vi "initalize 4200(SubVI).vi"(0 "簇":T4={"initialize"=enum."SR830", "6221"={"6221 Resource"="GPIB0::24::INSTR", "Delta status"=FALSE, "电流|RMS(A)"=0.0}, "SR830+6221"={"source"=0, "Current(A)"=0.0, "阻抗(Ohm)"=0.0, "SR830 1"=FALSE, "SR830 2"=FALSE, "SR830 3"=FALSE, "SR830 4"=FALSE, "VISA 1"="", "VISA 2"="", "VISA 3"="", "VISA 4"="", "Reserve 1"=0, "Reserve 2"=-1, "Reserve 3"=-1, "Reserve 4"=-1, "Sensitivity 1"=-1, "Sensitivity 2"=-1, "Sensitivity 3"=-1, "Sensitivity 4"=-1, "量程入 1"=0, "量程入 2"=0, "量程入 3"=0, "量程入 4"=0}, "2400"={"2400"=FALSE, "VISA"="", "Output Level (0)"=1e-05, "Compliance  Level (0.1)"=10.0, "ch"=[]}, "ch"={"ch"=[], "current"=[], "change?"=[], "holding current\nwhen change ch?"=FALSE, "current offset"=[]}, "Instrument"={"limit"={"Field limit"=0.0, "Field rate limit"=0.0, "Temp limit"=0.0, "Temp low limit"=0.0, "Temp rate limit "=0.0}, "genarl"={"行数"=refnum, "编辑列表框？"=refnum, "列表框"=refnum, "camg 振荡状态"=refnum, "Aborting"=refnum, "数据文件"=refnum, "warning"=refnum, "vi路径"="", "Instrument Type"=enum."PPMS-Rotate"}, "cmag"={"TM620"="TCPIP0::192.168.1.5::4266::SOCKET", "M24C Resource"="GPIB0::24::INSTR", "4G supply"="", "Temp Status 24C"=refnum, "Temp"=refnum, "9T信号"=refnum, "4g supply status"=refnum, "in-plane"="", "out-plane"="", "in-plane signal"=FALSE, "out-plane signal"=FALSE, "in plane 信号"=refnum, "pzt volt"=refnum, "camg Rate"=refnum}, "lengtou2"={"750 visa"="", "750 rotate"="", "semaphore 340"=refnum, "semaphore 750"=refnum, "750 field status"=refnum, "Input (0:A) 340"=0, "340 Resource"="GPIB0::14::INSTR", "340 Status"=refnum, "Input (0:B) 340"=1, "Loop (0: 1)"=0, "Loop (1: 1)"=0, "TCP master instance"=refnum}, "lengtou"={"TCP master instance"=refnum, "335 Status"=refnum, "335 Resource "="GPIB0::24::INSTR", "Input (0:A) 335"=0, "Input (0:B) 335"=1, "Heater Output (1:1) 335"=1, "semaphore 335"=refnum}, "325 for test"={"quantum design"=refnum, "semaphore 325"=refnum, "325 Resource "="GPIB0::13::INSTR", "Input (0:A) 325"=0, "Heater Output (1:1) 325"=1, "325 Status"=refnum}}, "2614B"={"2614B chA"=FALSE, "2614B chB"=FALSE, "VISA"=""}, "33522b"={"33522b resource name"="GPIB0::16::INSTR", "零电压"=0.0, "最大电压"=148.0, "间隔"=4.0, "最小电压"=-48.0, "loop"=0.0, "压电陶瓷电压(Vpp)"=0.0}, "gating type"=enum."2614(daul)", "层数"=0, "行数"=0, "是否处理"=[], "current 2"=[], "StrainCell"={"RP100 resource name"="GPIB0::16::INSTR", "E4980 resource name"="GPIB0::16::INSTR", "RP100 Reset ?(True)"=TRUE, "Voltage1(V)"=0.0, "Voltage2(V)"=148.0, "interval"=4.0, "slew(V/s)"=-48.0}} {"Instrument"."325 for test"."Heater Output (1:1) 325" items=["1"=1, "2"=2]; "Instrument"."325 for test"."Input (0:A) 325" items=["A", "B"]; "Instrument"."lengtou"."Heater Output (1:1) 335" items=["1"=1, "2"=2]; "Instrument"."lengtou"."Input (0:B) 335" items=["A", "B"]; "Instrument"."lengtou"."Input (0:A) 335" items=["A", "B"]; "Instrument"."lengtou2"."Loop (1: 1)" items=["1", "2"]; "Instrument"."lengtou2"."Loop (0: 1)" items=["1", "2"]; "Instrument"."lengtou2"."Input (0:B) 340" items=["A", "B", "C", "D"]; "Instrument"."lengtou2"."Input (0:A) 340" items=["A", "B", "C", "D"]; "SR830+6221"."Sensitivity 4" items=["量程每次测量会判定", "量程不变为设定值"]; "SR830+6221"."Sensitivity 3" items=["Auto Reserve"=-1, "High Reserve"=0, "Normal"=1, "Low Noise"=2]; "SR830+6221"."Sensitivity 1" items=["Auto Reserve"=-1, "High Reserve"=0, "Normal"=1, "Low Noise"=2]; "SR830+6221"."Sensitivity 2" items=["Auto Reserve"=-1, "High Reserve"=0, "Normal"=1, "Low Noise"=2]; "SR830+6221"."Reserve 4" items=["量程每次测量会判定", "量程不变为设定值"]; "SR830+6221"."Reserve 3" items=["Auto Reserve"=-1, "High Reserve"=0, "Normal"=1, "Low Noise"=2]; "SR830+6221"."Reserve 2" items=["Auto Reserve"=-1, "High Reserve"=0, "Normal"=1, "Low Noise"=2]; "SR830+6221"."Reserve 1" items=["Auto Reserve"=-1, "High Reserve"=0, "Normal"=1, "Low Noise"=2]; "SR830+6221"."source" items=["SR830 1", "SR830 2", "SR830 3", "SR830 4"]}, 2 "字符串":string) -> (7 "输出簇":T4={"initialize"=enum."SR830", "6221"={"6221 Resource"="GPIB0::24::INSTR", "Delta status"=FALSE, "电流|RMS(A)"=0.0}, "SR830+6221"={"source"=0, "Current(A)"=0.0, "阻抗(Ohm)"=0.0, "SR830 1"=FALSE, "SR830 2"=FALSE, "SR830 3"=FALSE, "SR830 4"=FALSE, "VISA 1"="", "VISA 2"="", "VISA 3"="", "VISA 4"="", "Reserve 1"=0, "Reserve 2"=-1, "Reserve 3"=-1, "Reserve 4"=-1, "Sensitivity 1"=-1, "Sensitivity 2"=-1, "Sensitivity 3"=-1, "Sensitivity 4"=-1, "量程入 1"=0, "量程入 2"=0, "量程入 3"=0, "量程入 4"=0}, "2400"={"2400"=FALSE, "VISA"="", "Output Level (0)"=1e-05, "Compliance  Level (0.1)"=10.0, "ch"=[]}, "ch"={"ch"=[], "current"=[], "change?"=[], "holding current\nwhen change ch?"=FALSE, "current offset"=[]}, "Instrument"={"limit"={"Field limit"=0.0, "Field rate limit"=0.0, "Temp limit"=0.0, "Temp low limit"=0.0, "Temp rate limit "=0.0}, "genarl"={"行数"=refnum, "编辑列表框？"=refnum, "列表框"=refnum, "camg 振荡状态"=refnum, "Aborting"=refnum, "数据文件"=refnum, "warning"=refnum, "vi路径"="", "Instrument Type"=enum."PPMS-Rotate"}, "cmag"={"TM620"="TCPIP0::192.168.1.5::4266::SOCKET", "M24C Resource"="GPIB0::24::INSTR", "4G supply"="", "Temp Status 24C"=refnum, "Temp"=refnum, "9T信号"=refnum, "4g supply status"=refnum, "in-plane"="", "out-plane"="", "in-plane signal"=FALSE, "out-plane signal"=FALSE, "in plane 信号"=refnum, "pzt volt"=refnum, "camg Rate"=refnum}, "lengtou2"={"750 visa"="", "750 rotate"="", "semaphore 340"=refnum, "semaphore 750"=refnum, "750 field status"=refnum, "Input (0:A) 340"=0, "340 Resource"="GPIB0::14::INSTR", "340 Status"=refnum, "Input (0:B) 340"=1, "Loop (0: 1)"=0, "Loop (1: 1)"=0, "TCP master instance"=refnum}, "lengtou"={"TCP master instance"=refnum, "335 Status"=refnum, "335 Resource "="GPIB0::24::INSTR", "Input (0:A) 335"=0, "Input (0:B) 335"=1, "Heater Output (1:1) 335"=1, "semaphore 335"=refnum}, "325 for test"={"quantum design"=refnum, "semaphore 325"=refnum, "325 Resource "="GPIB0::13::INSTR", "Input (0:A) 325"=0, "Heater Output (1:1) 325"=1, "325 Status"=refnum}}, "2614B"={"2614B chA"=FALSE, "2614B chB"=FALSE, "VISA"=""}, "33522b"={"33522b resource name"="GPIB0::16::INSTR", "零电压"=0.0, "最大电压"=148.0, "间隔"=4.0, "最小电压"=-48.0, "loop"=0.0, "压电陶瓷电压(Vpp)"=0.0}, "gating type"=enum."2614(daul)", "层数"=0, "行数"=0, "是否处理"=[], "current 2"=[], "StrainCell"={"RP100 resource name"="GPIB0::16::INSTR", "E4980 resource name"="GPIB0::16::INSTR", "RP100 Reset ?(True)"=TRUE, "Voltage1(V)"=0.0, "Voltage2(V)"=148.0, "interval"=4.0, "slew(V/s)"=-48.0}} {"Instrument"."325 for test"."Heater Output (1:1) 325" items=["1"=1, "2"=2]; "Instrument"."325 for test"."Input (0:A) 325" items=["A", "B"]; "Instrument"."lengtou"."Heater Output (1:1) 335" items=["1"=1, "2"=2]; "Instrument"."lengtou"."Input (0:B) 335" items=["A", "B"]; "Instrument"."lengtou"."Input (0:A) 335" items=["A", "B"]; "Instrument"."lengtou2"."Loop (1: 1)" items=["1", "2"]; "Instrument"."lengtou2"."Loop (0: 1)" items=["1", "2"]; "Instrument"."lengtou2"."Input (0:B) 340" items=["A", "B", "C", "D"]; "Instrument"."lengtou2"."Input (0:A) 340" items=["A", "B", "C", "D"]; "SR830+6221"."Sensitivity 4" items=["量程每次测量会判定", "量程不变为设定值"]; "SR830+6221"."Sensitivity 3" items=["Auto Reserve"=-1, "High Reserve"=0, "Normal"=1, "Low Noise"=2]; "SR830+6221"."Sensitivity 1" items=["Auto Reserve"=-1, "High Reserve"=0, "Normal"=1, "Low Noise"=2]; "SR830+6221"."Sensitivity 2" items=["Auto Reserve"=-1, "High Reserve"=0, "Normal"=1, "Low Noise"=2]; "SR830+6221"."Reserve 4" items=["量程每次测量会判定", "量程不变为设定值"]; "SR830+6221"."Reserve 3" items=["Auto Reserve"=-1, "High Reserve"=0, "Normal"=1, "Low Noise"=2]; "SR830+6221"."Reserve 2" items=["Auto Reserve"=-1, "High Reserve"=0, "Normal"=1, "Low Noise"=2]; "SR830+6221"."Reserve 1" items=["Auto Reserve"=-1, "High Reserve"=0, "Normal"=1, "Low Noise"=2]; "SR830+6221"."source" items=["SR830 1", "SR830 2", "SR830 3", "SR830 4"]})   [LabVIEW 2019, in "initialize.lvlib"]
uses:
  initialize.lvlib
  ctl/config.ctl
  <vilib>/NI/Modbus Library/API/Master/Modbus Master.lvclass
  ctl/initialize.ctl
  ctl/Instrument.ctl
  ctl/limit.ctl
  ctl/warning.ctl
  ctl/Instrument Type.ctl
  ctl/335 state.ctl
  ctl/9T mag field stauts.ctl
  C:/Users/fuyang/Desktop/postdoctor/labview/labview-measure/lib/QDInstrument.dll
  lib/QDInstrument.dll
  ctl/Gating type.ctl
panel:
  out "Name array 2":string[](array[string])
  in  "SMU2(Ryx) Setup":T1={"Enable"=TRUE, "Source Mode"=enum."Voltage Source", "Compliance (V/A)"=0.1, "Source V/I (V/A)"=0.0, "Current Measurement Range\n(Limited Auto)"=9} {"Current Measurement Range\n(Limited Auto)" items=["1 pA (pre-Amp only)", "10 pA (pre-Amp only)", "100 pA (pre-Amp only)", "1 nA", "10 nA", "100 nA", "1 uA", "10 uA", "100 uA", "1 mA", "10 mA", "100 mA", "1 A (4210-SMU only)"]; "Source V/I (V/A)" min=-100.0 max=100.0 step=0.0001 format="%^.2e"; "Compliance (V/A)" min=-210.0 max=210.0 format="%_3e"}
  in  "SMU1(Rxx) Setup":T1={"Enable"=TRUE, "Source Mode"=enum."Voltage Source", "Compliance (V/A)"=0.1, "Source V/I (V/A)"=0.0, "Current Measurement Range\n(Limited Auto)"=9} {"Current Measurement Range\n(Limited Auto)" items=["1 pA (pre-Amp only)", "10 pA (pre-Amp only)", "100 pA (pre-Amp only)", "1 nA", "10 nA", "100 nA", "1 uA", "10 uA", "100 uA", "1 mA", "10 mA", "100 mA", "1 A (4210-SMU only)"]; "Source V/I (V/A)" min=-100.0 max=100.0 step=0.0001 format="%^.2e"; "Compliance (V/A)" min=-210.0 max=210.0 format="%_3e"}
  in  "Integration Time":i16(slide)=2 min=1 max=3 step=1 scale=1.0..3.0
  out "Name array":string[](array[string])
  out "SMU1 status":T2
  out "4200 GPIB address out":string="1::17"
  out "error out":errorcluster
  in  "error in":errorcluster
  out "Instrument ID":string
  in  "4200 GPIB address in":string="1:17"
  in  "Sampling Mode Timing":T3={"Wait Time"=0.0, "Interval"=0.1, "No. of Readings"=5} {"No. of Readings" min=1 max=4097 step=1; "Interval" min=0.0 max=10.0 step=0.001 format="%.2g"; "Wait Time" min=0.0 max=100.0 step=0.1 format="%.3g"}
  out "SMU2 status":T2
  # "Please make sure KI 4200 is in Normal Mode (under KCON).\nStart KXCI before running this VI."
  # "Hold up start of test (s)"
  # "Time between measurements(s)"
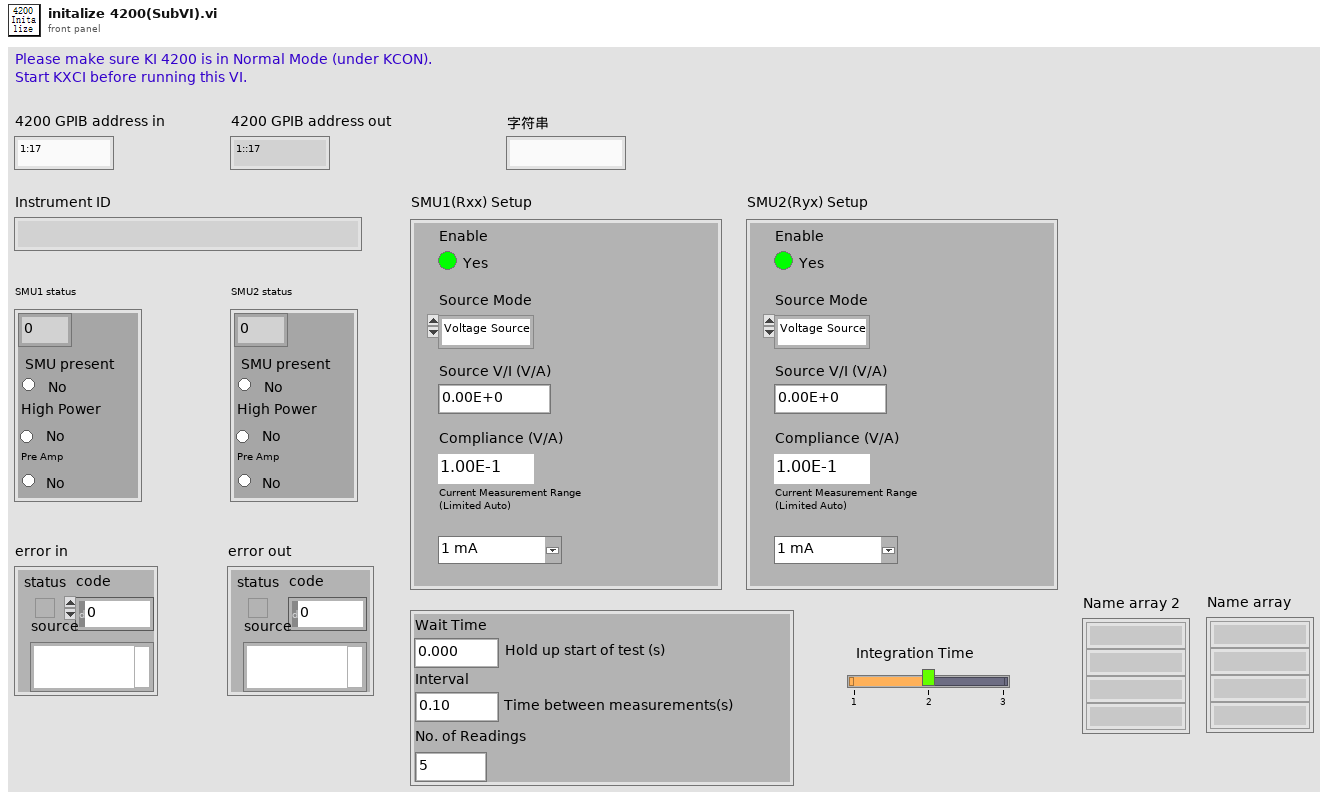
[diagram p1: front panel]
types:
  T1 = cluster{"Enable":bool, "Source Mode":enum16{"Voltage Source", "Current Source", "Common"}, "Compliance (V/A)":dbl, "Source V/I (V/A)":dbl, "Current Measurement Range\n(Limited Auto)":u16}
  T2 = cluster{"SMU No.":i32, "SMU present":bool, "High Power":bool, "Pre Amp":bool}
  T3 = cluster{"Wait Time":dbl, "Interval":dbl, "No. of Readings":i16}
  T4 = typedef "config.ctl" = cluster{"initialize":T5, "6221":cluster{"6221 Resource":refnum<visa-resource-name>, "Delta status":bool, "电流|RMS(A)":dbl}, "SR830+6221":cluster{"source":u16, "Current(A)":dbl, "阻抗(Ohm)":dbl, "SR830 1":bool, "SR830 2":bool, "SR830 3":bool, "SR830 4":bool, "VISA 1":refnum<visa-resource-name>, "VISA 2":refnum<visa-resource-name>, "VISA 3":refnum<visa-resource-name>, "VISA 4":refnum<visa-resource-name>, "Reserve 1":i16, "Reserve 2":i16, "Reserve 3":i16, "Reserve 4":i16, "Sensitivity 1":i16, "Sensitivity 2":i16, "Sensitivity 3":i16, "Sensitivity 4":i16, "量程入 1":i32, "量程入 2":i32, "量程入 3":i32, "量程入 4":i32}, "2400":cluster{"2400":bool, "VISA":refnum<visa-resource-name>, "Output Level (0)":dbl, "Compliance  Level (0.1)":dbl, "ch":i32[]}, "ch":cluster{"ch":i32[], "current":dbl[], "change?":bool[], "holding current\nwhen change ch?":bool, "current offset":dbl[]}, "Instrument":T6, "2614B":cluster{"2614B chA":bool, "2614B chB":bool, "VISA":refnum<visa-resource-name>}, "33522b":cluster{"33522b resource name":refnum<visa-resource-name>, "零电压":dbl, "最大电压":dbl, "间隔":dbl, "最小电压":dbl, "loop":dbl, "压电陶瓷电压(Vpp)":dbl}, "gating type":T10, "层数":i32, "行数":i32, "是否处理":bool[], "current 2":dbl[], "StrainCell":cluster{"RP100 resource name":refnum<visa-resource-name>, "E4980 resource name":refnum<visa-resource-name>, "RP100 Reset ?(True)":bool, "Voltage1(V)":dbl, "Voltage2(V)":dbl, "interval":dbl, "slew(V/s)":dbl}}
  T5 = typedef "initialize.ctl" = enum16{"SR830", "keithley6221-SR830", "Delta", "Delta-tunnelling", "keithley6221-2182-DC", "PZT", "StrainCell", "4200"}
  T6 = typedef "Instrument.ctl" = cluster{"limit":T7, "genarl":cluster{"行数":refnum<vi>, "编辑列表框？":refnum<vi>, "列表框":refnum<vi>, "camg 振荡状态":refnum<vi>, "Aborting":refnum<vi>, "数据文件":refnum<vi>, "warning":refnum<vi>, "vi路径":string, "Instrument Type":T8}, "cmag":cluster{"TM620":refnum<visa-resource-name>, "M24C Resource":refnum<visa-resource-name>, "4G supply":refnum<visa-resource-name>, "Temp Status 24C":refnum<vi>, "Temp":refnum<vi>, "9T信号":T9, "4g supply status":refnum<vi>, "in-plane":refnum<visa-resource-name>, "out-plane":refnum<visa-resource-name>, "in-plane signal":bool, "out-plane signal":bool, "in plane 信号":T9, "pzt volt":refnum<vi>, "camg Rate":refnum<vi>}, "lengtou2":cluster{"750 visa":refnum<visa-resource-name>, "750 rotate":refnum<visa-resource-name>, "semaphore 340":T9, "semaphore 750":T9, "750 field status":refnum<vi>, "Input (0:A) 340":u16, "340 Resource":refnum<visa-resource-name>, "340 Status":refnum<vi>, "Input (0:B) 340":u16, "Loop (0: 1)":u16, "Loop (1: 1)":u16, "TCP master instance":refnum<class "Modbus Master.lvclass">}, "lengtou":cluster{"TCP master instance":refnum<class "Modbus Master.lvclass">, "335 Status":refnum<vi>, "335 Resource ":refnum<visa-resource-name>, "Input (0:A) 335":u16, "Input (0:B) 335":u16, "Heater Output (1:1) 335":u16, "semaphore 335":T9}, "325 for test":cluster{"quantum design":refnum<k24>, "semaphore 325":T9, "325 Resource ":refnum<visa-resource-name>, "Input (0:A) 325":u16, "Heater Output (1:1) 325":u16, "325 Status":refnum<vi>}}
  T7 = typedef "limit.ctl" = cluster{"Field limit":dbl, "Field rate limit":dbl, "Temp limit":dbl, "Temp low limit":dbl, "Temp rate limit ":dbl}
  T8 = typedef "Instrument Type.ctl" = enum16{"PPMS", "VersaLab", "DynaCool", "SVSM", "PPMS-Rotate", "Lakeshore335", "lengtou2", "9T mag old", "9T cmag", "9T cmag DAC", "9T cmag rotate", "test"}
  T9 = typedef "Semaphore RefNum" = refnum<k1>
  T10 = typedef "Gating type.ctl" = enum32{"null", "2614(daul)", "2400", "6517B"}
  T11 = enum16{"SMU 1", "SMU 2", "SMU 3", "SMU 4", "SMU 5", "SMU 6", "SMU 7", "SMU 8"}
  T12 = enum16{"Sweep (master)", "Step (master)", "Fixed", "Sweep (slave)"}
  T13 = enum16{"Voltage Source", "Current Source", "Common"}
  T14 = cluster{"Enable":bool, "Source Mode":enum16{"Voltage Source", "Current Source", "Common"}, "Source Function":enum16{"Sweep (master)", "Step (master)", "Fixed", "Sweep (slave)"}, "I name":string, "I name":string, "Compliance (V/A)":dbl, "Source V/I (V/A)":dbl, "Current Measurement Range\n(Limited Auto)":u16}
  T15 = cluster{"error":bool, "code":i32, "source":string}
  T16 = cluster{"Delay factor":dbl, "Delay factor":dbl, "Delay factor":dbl, "Use Custom?":bool}
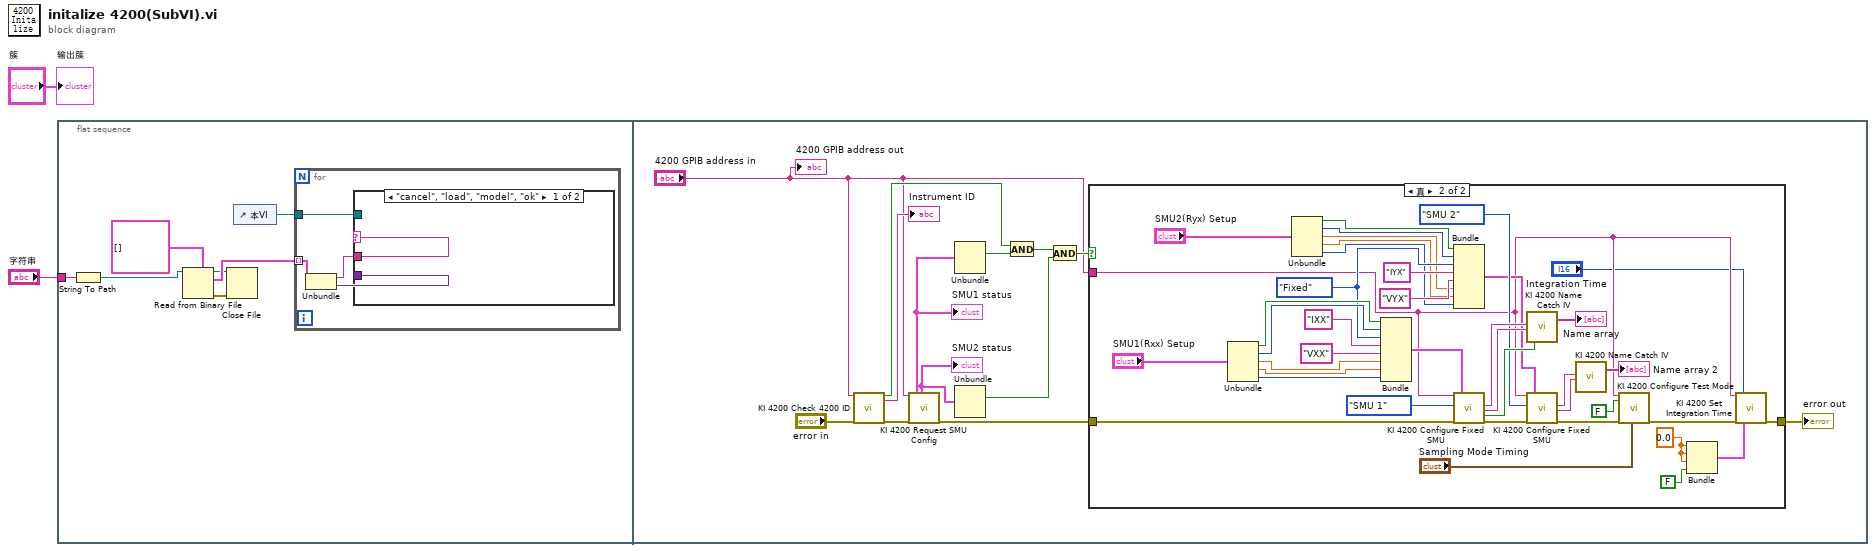
[diagram p0: block diagram]
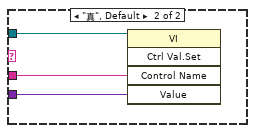
[diagram p2: hidden frame]
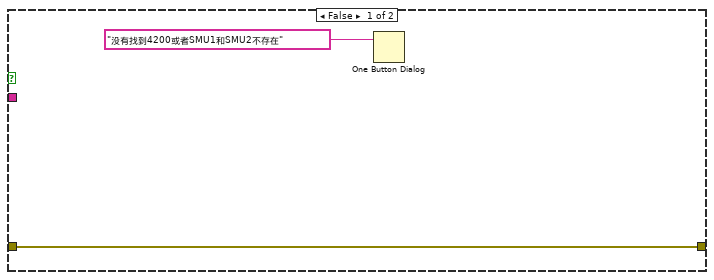
[diagram p3: hidden frame]
diagram:
  n1 = flat-sequence {
    tunnel: "字符串" -> [w3]
    frame #0 {
      n2 = String To Path(string=w3) -> (path=w8:path)
      n3 = Read from Binary File(5:cluster{"Name":string, "Variant Data":variant}[] [] ("控件值:获取全部"), 11:w8) -> (0:w4:errorcluster, 2:w6:cluster{"Name":string, "Variant Data":variant}[], 3:w5:refnum<file>)  [unwired: 4 in, 1 out]
      n4 = Close File(refnum=w5, error in=w4) -> ()  [unwired: 2 out]
      n5 = control-ref of="本VI"() -> (w9:refnum<vi>)
      n6 = for {
        tunnel: w6 -> [w13] mode=indexing
        tunnel: w9 -> [w12]
        n7 = Unbundle(w13) -> ("Name"=w10:string, "Variant Data"=w11:variant)
        n8 = case shown="\"cancel\", \"load\", \"model\", \"ok\"" w10 {
          tunnel: w12 -> [_ w16]
          tunnel: w10 -> [_ w15]
          tunnel: w11 -> [_ w14]
          frame "cancel", "load", "model", "ok" {
          }
          frame "真", Default {
            n9 = invoke class="VI" method="Ctrl Val.Set"(reference=w16, "Control Name"=w15, "Value"=w14) -> ()  [unwired: 2 in, 5 out]
          }
        }
      }
    }
    frame #1 {
      n10 = call "KI 4200 Check 4200 ID.vi"("GPIB add"="4200 GPIB address in", "error in"="error in") -> ("Is 4200?"=w24:bool, "Instr ID"=→"Instrument ID":string, "error out"=w23:errorcluster)  [unwired: 13 in, 2 out]
      n11 = call "KI 4200 Request SMU Config.vi"("GPIB add"="4200 GPIB address in", "error in"=w23) -> ("SMU1 status"=w26:T2, "SMU 2 status"=w27:T2, "error out"=w19:errorcluster)  [unwired: 8 in, 7 out]
      "SMU2 status" <- w27
      "SMU1 status" <- w26
      n12 = Unbundle(w26) -> ("SMU present"=w25:bool)  [unwired: 3 out]
      n13 = Unbundle(w27) -> ("SMU present"=w29:bool)  [unwired: 3 out]
      n14 = And(x=w24, y=w25) -> (x .and. y?=w28:bool)
      n15 = And(x=w28, y=w29) -> (x .and. y?=w20:bool)
      n16 = case shown="真" w20 {
        tunnel: w19 -> [w30 w65]
        tunnel: [w30 w32] -> w18
        tunnel: "4200 GPIB address in" -> [_ w39]
        frame False {
          n17 = One Button Dialog(message="没有找到4200或者SMU1和SMU2不存在") -> ()  [unwired: 1 in, 1 out]
        }
        frame True {
          w35 = 0.0 ("Delay factor")
          w51 = T12."Fixed" ("Source Function")
          n18 = Unbundle("SMU1(Rxx) Setup") -> ("Enable"=w61:bool, "Source Mode"=w60:T13, "Compliance (V/A)"=w50:dbl, "Source V/I (V/A)"=w49:dbl, "Current Measurement Range\n(Limited Auto)"=w48:u16)
          n19 = Unbundle("SMU2(Ryx) Setup") -> ("Enable"=w55:bool, "Source Mode"=w54:T13, "Compliance (V/A)"=w45:dbl, "Source V/I (V/A)"=w46:dbl, "Current Measurement Range\n(Limited Auto)"=w47:u16)
          n20 = Bundle("Enable"=w61, "Source Mode"=w60, "Source Function"=w51, "I name"="IXX", "I name"="VXX", "Compliance (V/A)"=w50, "Source V/I (V/A)"=w49, "Current Measurement Range\n(Limited Auto)"=w48) -> (w71:T14)  [unwired: 1 in]
          n21 = Bundle("Enable"=w55, "Source Mode"=w54, "Source Function"=w51, "I name"="IYX", "I name"="VYX", "Compliance (V/A)"=w45, "Source V/I (V/A)"=w46, "Current Measurement Range\n(Limited Auto)"=w47) -> (w57:T14)  [unwired: 1 in]
          n22 = call "KI 4200 Configure Fixed SMU .vi"("GPIB address"=w39, "channel"=T11."SMU 1", "error in"=w65, "Fixed Source Setup"=w71) -> ("I name"=w68:string, "V name"=w69:string, "Enable"=w67:bool, "error out"=w63:T15)  [unwired: 11 in, 1 out]
          n23 = call "KI 4200 Name Catch IV.vi"("I name"=w68, "V name"=w69, "Enable"=w67) -> ("Name array"=→"Name array":string[])  [unwired: 15 in, 1 out]
          n24 = call "KI 4200 Configure Fixed SMU .vi"("GPIB address"=w39, "channel"=T11."SMU 2", "error in"=w63, "Fixed Source Setup"=w57) -> ("I name"=w44:string, "V name"=w43:string, "error out"=w41:T15)  [unwired: 11 in, 2 out]
          n25 = call "KI 4200 Name Catch IV.vi"("I name"=w44, "V name"=w43) -> ("Name array"=→"Name array 2":string[])  [unwired: 16 in, 1 out]
          n26 = call "KI 4200 Configure Test Mode .vi"("GPIB address"=w39, "Sweeping"=FALSE, "error in (no error)"=w41, "Sampling Mode Timing"="Sampling Mode Timing") -> ("error out"=w40:errorcluster)  [unwired: 15 in]
          n27 = Bundle("Delay factor"=w35, "Delay factor"=w35, "Delay factor"=w35, "Use Custom?"=FALSE) -> (w33:T16)  [unwired: 1 in]
          n28 = call "KI 4200 Set Integration Time.vi"("GPIB address"=w39, "error in"=w40, "Integration Time"="Integration Time", "Custom Integration Settings"=w33) -> ("error out"=w32:T15)  [unwired: 13 in, 2 out]
        }
      }
      "error out" <- w18
      "4200 GPIB address out" <- "4200 GPIB address in"
    }
  }
  "输出簇" <- "簇"
